vi "Parse Data.vi"(9 "Read Buffer":string, 10 "Data Length":i32) -> (2 "Output Data Array":dbl[](array[numeric]))   [LabVIEW 2014, in "Agilent U2000 Series.lvlib"]
doc: "Parses IEEE 488.2 arbitrary block program data format to 32-bit floating point numbers."
uses:
  Agilent U2000 Series.lvlib
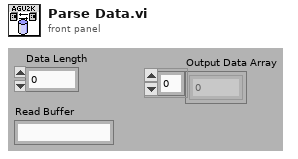
[diagram p1: front panel]
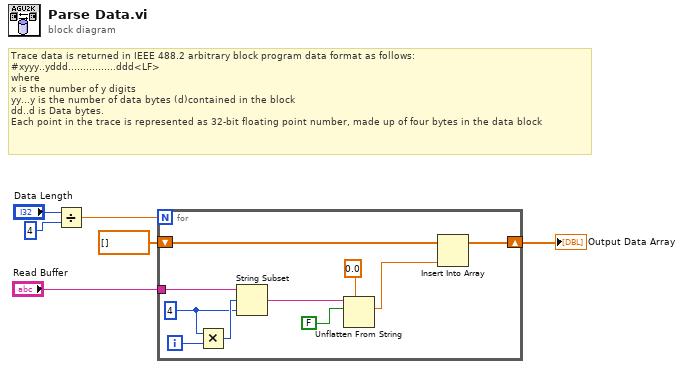
[diagram p0: block diagram]
diagram:
  # "Trace data is returned in IEEE 488.2 arbitrary block program data format as follows:\n#xyyy..yddd................ddd<LF>\nwhere \nx is the number of y digits\nyy...y is the number of data bytes (d)contained in the block\ndd..d is Data bytes. \nEach point in the trace is represented as 32-bit floating point number, made up of four bytes in the data block"
  n1 = Divide(x="Data Length", y=4) -> (x/y=w3:dbl)
  n2 = for {
    N: w3 -> [_]
    tunnel: "Read Buffer" -> [w16]
    shift-right: [w11] -> w5
    shift-left: dbl[] [] -> [w12]
    i -> [w15]
    w13 = 4 ("x")
    n3 = Multiply(x=w13, y=w15) -> (x*y=w14:i32)
    n4 = String Subset(string=w16, offset (0)=w14, length (rest)=w13) -> (substring=w10:string)
    n5 = Unflatten From String(type=sgl 0.0, binary string=w10, data includes array or string size? (T)=FALSE) -> (value=w9:sgl)  [unwired: 2 in, 2 out]
    n6 = Insert Into Array(array=w12, new element=w9) -> (w11:dbl[])  [unwired: 1 in]
  }
  "Output Data Array" <- w5
